vi "Initialize.vi"(8 "error in (no error)":errorcluster, 10 "attenuation":dbl=53.2) -> (0 "error out":errorcluster, 3 "Power Meter out":refnum<class "Power Meter.lvclass">)   [LabVIEW 2018, in "Power Meter.lvlib" / "Power Meter.lvclass"]
uses:
  Power Meter.lvclass
  Power Meter.lvclass/Power Meter.ctl
  Power Meter.lvlib
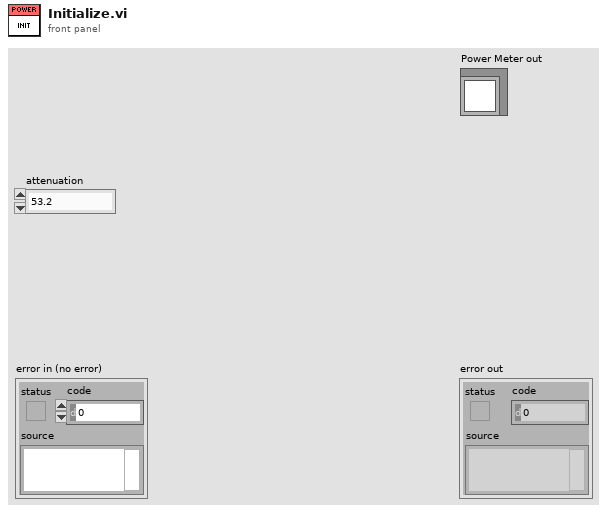
[diagram p1: front panel]
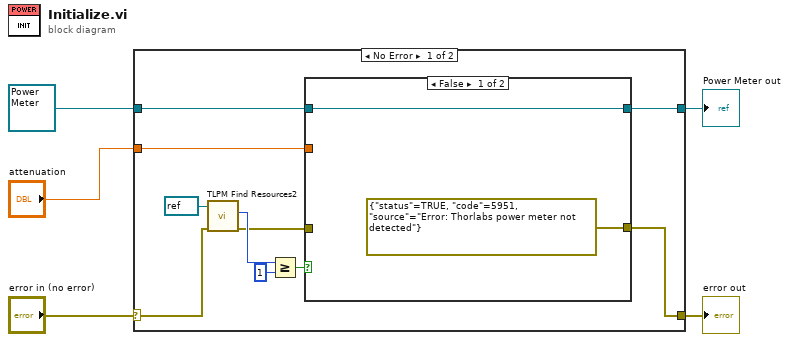
[diagram p0: block diagram]
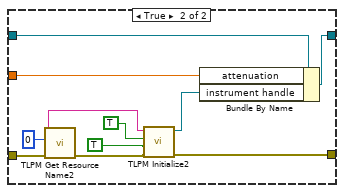
[diagram p2: hidden frame]
diagram:
  n1 = case shown="No Error" "error in (no error)" {
    selector: "error in (no error)" -> [w10 w30]
    tunnel: [w9 w30] -> w4
    tunnel: [w8 w29] -> w2
    tunnel: refnum<class "Power Meter.lvclass"> refnum ("Power Meter in") -> [w7 w29]
    tunnel: "attenuation" -> [w6 _]
    frame No Error {
      n2 = call "TLPM Find Resources2.vi"("error in (no error)"=w10, "instrument handle"=refnum<visa-resource-name> refnum) -> ("error out"=w14:errorcluster, "Resource Count"=w15:u32)  [unwired: 7 in, 1 out]
      n3 = Greater Or Equal?(x=w15, y=u32 1) -> (x >= y?=w13:bool)
      n4 = case shown="False" w13 {
        tunnel: w14 -> [_ w28]
        tunnel: [errorcluster {"status"=TRUE, "code"=5951, "source"="Error: Thorlabs power meter not detected"} ("error constant") w25] -> w9
        tunnel: [w16 w19] -> w8
        tunnel: w7 -> [w16 w20]
        tunnel: w6 -> [_ w21]
        frame False {
        }
        frame True {
          n5 = call "TLPM Get Resource Name2.vi"("error in (no error)"=w28, "Index (0)"=u32 0 ("Device Index")) -> ("error out"=w26:errorcluster, "Resource Name"=w22:string)  [unwired: 7 in, 1 out]
          n6 = call "TLPM Initialize2.vi"("error in (no error)"=w26, "Reset Device (Reset Device)"=TRUE ("ID Query (Do Query)"), "ID Query (Do Query)"=TRUE, "resource name"=w22) -> ("error out"=w25:errorcluster, "instrument handle out"=w18:refnum<visa-resource-name>)  [unwired: 6 in]
          n7 = Bundle By Name(cluster=w20, "attenuation"=w21, "instrument handle"=w18) -> (w19:refnum<class "Power Meter.lvclass">)
        }
      }
    }
    frame Error {
    }
  }
  "error out" <- w4
  "Power Meter out" <- w2
